vi "TalonMotionMagic.vi"(0 "xMotorControlDevRef":T1={"DeviceStatus"={"status"=FALSE, "code"=0, "source"=""}, "Type"=enum."PWM", "PWM"={"PWM Channel"=enum."Invalid", "DeadBand"={"Name"="", "maxPositivePwm"=0, "minPositivePwm"=0, "centerPwm"=0, "maxNegativePwm"=0, "minNegativePwm"=0, "angularRange"=0}}, "CAN"={"Device Number"=0, "SetOutput VI Ref"=variant, "GetOutput VI Ref"=variant, "Enable VI Ref"=variant, "Disable VI Ref"=variant, "Data"=variant}, "Invert"=FALSE, "DIO PWM"={"PWM \"Enable\" Channel"=enum."Invalid", "DIOChannel"=enum."Invalid", "PWM Rate"=0.0}}, 1 "Boolean Value Inputs":T7, 2 "Numeric Value Inputs":T6, 3 "error in":errorcluster) -> (5 "PhoenixMotorControlDevRef":T1={"DeviceStatus"={"status"=FALSE, "code"=0, "source"=""}, "Type"=enum."PWM", "PWM"={"PWM Channel"=enum."Invalid", "DeadBand"={"Name"="", "maxPositivePwm"=0, "minPositivePwm"=0, "centerPwm"=0, "maxNegativePwm"=0, "minNegativePwm"=0, "angularRange"=0}}, "CAN"={"Device Number"=0, "SetOutput VI Ref"=variant(enum8{"Percent VBus", "Current", "Speed", "Position", "Voltage"} enum."Percent VBus"), "GetOutput VI Ref"=variant(refnum<k1> refnum), "Enable VI Ref"=variant(dbl 12.0), "Disable VI Ref"=variant(enum8{"Percent VBus", "Speed", "Position", "Slave", "Unchanged / Invalid", "Voltage Compensation", "Current", "Motion Profile"} enum."Percent VBus"), "Data"=variant}, "Invert"=FALSE, "DIO PWM"={"PWM \"Enable\" Channel"=enum."Invalid", "DIOChannel"=enum."Invalid", "PWM Rate"=0.0}}, 6 "Graph Output":cluster{"Hood Setpoint":dbl, dbl}, 7 "error out":errorcluster)   [LabVIEW 2020]
uses:
  <vilib>/Rock Robotics/WPI/MotorControl/WPI_MotorControlDeviceRef.ctl
  <vilib>/Rock Robotics/WPI/MotorControl/WPI_MotorControlType.ctl
  <vilib>/Rock Robotics/SystemInterfaces/DIO/FPGA_DIOPWMChannel.ctl
  <vilib>/Rock Robotics/WPI/PWM/WPI_PWMDeadband.ctl
  <vilib>/Rock Robotics/SystemInterfaces/DIO/FPGA_DIOChannel.ctl
  <vilib>/Rock Robotics/WPI/ThirdParty/Phoenix-LabVIEW/Motor Controller/Controls/CTRE_Phoenix_MotorControl_ControlMode.ctl
  <vilib>/Rock Robotics/WPI/ThirdParty/Phoenix-LabVIEW/Motor Controller/Get/CTRE_Phoenix_MotorController_GetSelectedSensorData.vi
  TitanLib/Lib/TitanLib.lvlib
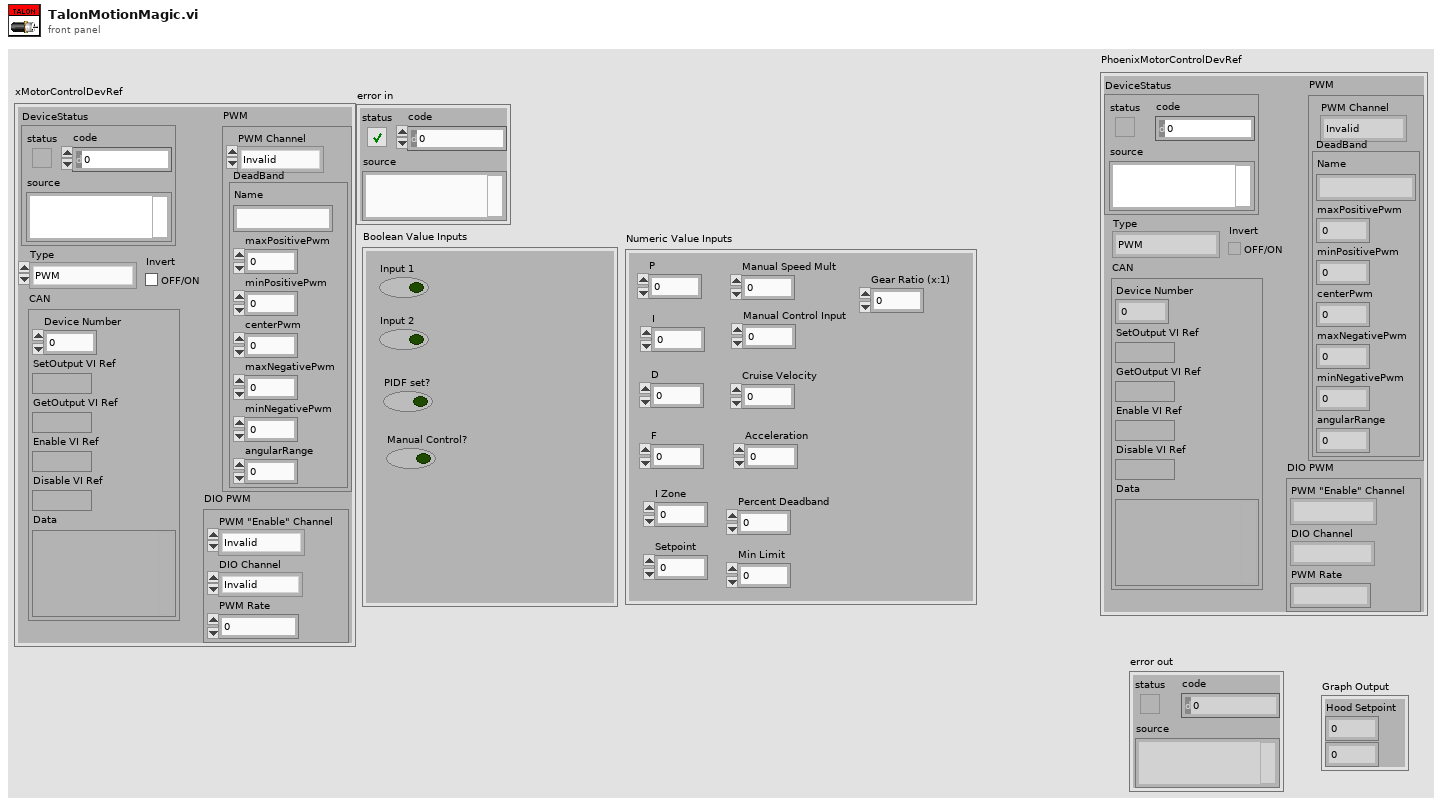
[diagram p1: front panel]
types:
  T1 = typedef "WPI_MotorControlDeviceRef.ctl" = cluster{"DeviceStatus":errorcluster, "Type":T2, "PWM":cluster{"PWM Channel":T3, "DeadBand":T4}, "CAN":cluster{"Device Number":u8, "SetOutput VI Ref":variant, "GetOutput VI Ref":variant, "Enable VI Ref":variant, "Disable VI Ref":variant, "Data":variant}, "Invert":bool, "DIO PWM":cluster{"PWM \"Enable\" Channel":T3, "DIOChannel":T5, "PWM Rate":dbl}}
  T2 = typedef "WPI_MotorControlType.ctl" = enum16{"PWM", "CAN", "DIO PWM"}
  T3 = typedef "FPGA_DIOPWMChannel.ctl" = enum8{"PWM 0", "PWM 1", "PWM 2", "PWM 3", "PWM 4", "PWM 5", "PWM 6", "PWM 7", "PWM 8", "PWM 9", "PWM MXP 0", "PWM MXP 1", "PWM MXP 2", "PWM MXP 3", "PWM MXP 4", "PWM MXP 5", "PWM MXP 6", "PWM MXP 7", "PWM MXP 8", "PWM MXP 9", "Invalid"}
  T4 = typedef "WPI_PWMDeadband.ctl" = cluster{"Name":string, "maxPositivePwm":i32, "minPositivePwm":i32, "centerPwm":i32, "maxNegativePwm":i32, "minNegativePwm":i32, "angularRange":u16}
  T5 = typedef "FPGA_DIOChannel.ctl" = enum8{"DIO 0", "DIO 1", "DIO 2", "DIO 3", "DIO 4", "DIO 5", "DIO 6", "DIO 7", "DIO 8", "DIO 9", "DIO MXP 0", "DIO MXP 1", "DIO MXP 2", "DIO MXP 3", "DIO MXP 4", "DIO MXP 5", "DIO MXP 6", "DIO MXP 7", "DIO MXP 8", "DIO MXP 9", "DIO MXP 10", "DIO MXP 11", "DIO MXP 12", "DIO MXP 13", "DIO MXP 14", "DIO MXP 15", "SPI Port CS1", "SPI Port CS2", "SPI Port CS3", "SPI Port MISO", "SPI Port MOSI", "Invalid"}
  T6 = cluster{"P":dbl, "I":dbl, "D":dbl, "F":dbl, "I Zone":dbl, "Setpoint":dbl, "Manual Speed Mult":dbl, "Manual Control Input":dbl, "Cruise Velocity":i32, "Acceleration":i32, "Percent Deadband":dbl, "Min Limit":dbl, "Gear Ratio (x:1)":dbl}
  T7 = cluster{"Input 1":bool, "Input 2":bool, "PIDF set?":bool, "Manual Control?":bool}
  T8 = typedef "CTRE_Phoenix_MotorControl_ControlMode.ctl" = u16
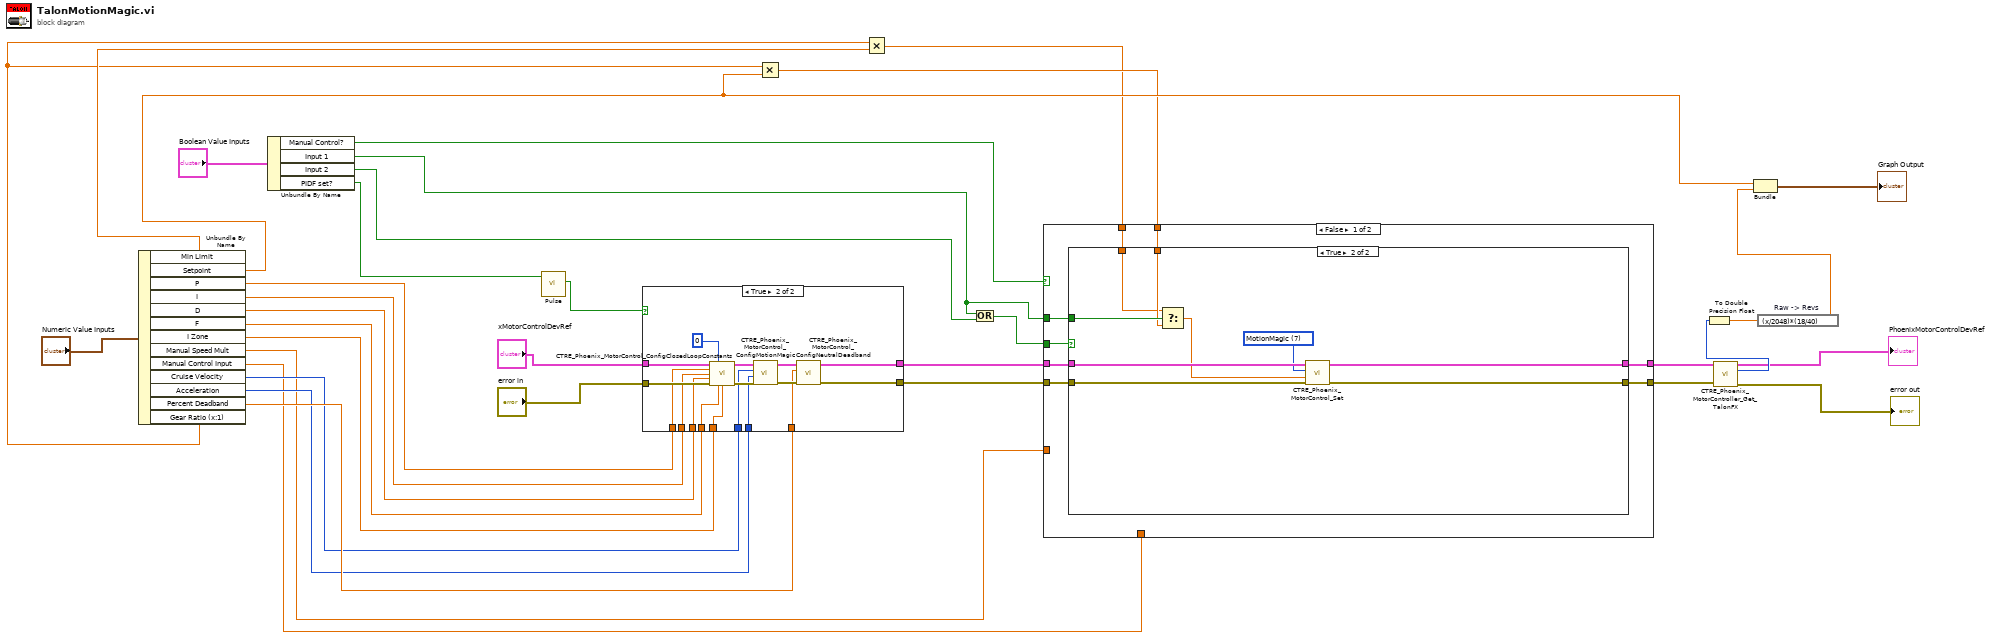
[diagram p0: block diagram]
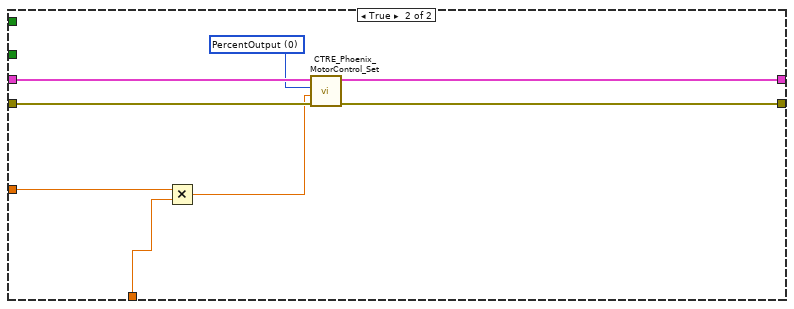
[diagram p3: hidden frame]
diagram:
  n1 = Unbundle By Name("Numeric Value Inputs") -> ("Min Limit"=w4:dbl, "Setpoint"=w5:dbl, "P"=w17:dbl, "I"=w16:dbl, "D"=w15:dbl, "F"=w14:dbl, "I Zone"=w13:dbl, "Manual Speed Mult"=w9:dbl, "Manual Control Input"=w8:dbl, "Cruise Velocity"=w11:i32, "Acceleration"=w10:i32, "Percent Deadband"=w12:dbl, "Gear Ratio (x:1)"=w3:dbl)
  n2 = Unbundle By Name("Boolean Value Inputs") -> ("Manual Control?"=w19:bool, "Input 1"=w20:bool, "Input 2"=w21:bool, "PIDF set?"=w22:bool)
  n3 = call "Pulse.vi"("Input"=w22) -> ("Output"=w26:bool)  [unwired: 10 in]
  n4 = case shown="True" w26 {
    tunnel: "xMotorControlDevRef" -> [w37 w54]
    tunnel: "error in" -> [w36 w53]
    tunnel: w17 -> [_ w52]
    tunnel: w16 -> [_ w51]
    tunnel: w15 -> [_ w50]
    tunnel: w14 -> [_ w49]
    tunnel: w13 -> [_ w48]
    tunnel: w11 -> [_ w45]
    tunnel: w10 -> [_ w44]
    tunnel: w12 -> [_ w41]
    tunnel: [w37 w40] -> w27
    tunnel: [w36 w39] -> w28
    frame False {
    }
    frame True {
      n5 = call <vilib>:"CTRE_Phoenix_MotorControl_ConfigClosedLoopConstants.vi"("PhoenixMotorControlDevRef"=w54, "slotIdx"=0, "P"=w52, "I"=w51, "D"=w50, "error in (no error)"=w53, "F"=w49, "I Zone"=w48) -> ("PhoenixMotorControlDevRef"=w46:T1, "error out"=w47:errorcluster)  [unwired: 6 in]
      n6 = call <vilib>:"CTRE_Phoenix_MotorControl_ConfigMotionMagic.vi"("error in (no error)"=w47, "Acceleration"=w44, "Cruise Velocity"=w45, "PhoenixMotorControlDevRef"=w46) -> ("error out"=w43:errorcluster, "PhoenixMotorControlDevRef"=w42:T1)  [unwired: 6 in]
      n7 = call <vilib>:"CTRE_Phoenix_MotorControl_ConfigNeutralDeadband.vi"("error in (no error)"=w43, "Percent Deadband"=w41, "PhoenixMotorControlDevRef"=w42) -> ("error out"=w39:errorcluster, "PhoenixMotorControlDevRef"=w40:T1)  [unwired: 7 in]
    }
  }
  n8 = Multiply(x=w3, y=w5) -> (x*y=w2:dbl)
  n9 = Multiply(x=w3, y=w4) -> (x*y=w1:dbl)
  n10 = Or(x=w20, y=w21) -> (x .or. y?=w29:bool)
  n11 = case shown="False" w19 {
    tunnel: w27 -> [w62 w81]
    tunnel: w28 -> [w61 w80]
    tunnel: w29 -> [w60 _]
    tunnel: w20 -> [w59 _]
    tunnel: w2 -> [w58 _]
    tunnel: w9 -> [_ w79]
    tunnel: [w57 w76] -> w30
    tunnel: [w56 w75] -> w31
    tunnel: w8 -> [_ w74]
    tunnel: w1 -> [w55 _]
    frame False {
      n12 = case shown="True" w60 {
        tunnel: w62 -> [w64 w73]
        tunnel: w61 -> [w63 w72]
        tunnel: w59 -> [_ w70]
        tunnel: w58 -> [_ w68]
        tunnel: [w64 w67] -> w57
        tunnel: [w63 w66] -> w56
        tunnel: w55 -> [_ w65]
        frame False {
        }
        frame True {
          w71 = T8 7 items=["PercentOutput"=0, "Position"=1, "Velocity"=2, "Current"=3, "Follower"=5, "MotionProfile"=6, "MotionMagic"=7, "MotionProfileArc"=10, "Disabled"=15] ("Control Mode")
          n13 = Select(t=w65, s=w70, f=w68) -> (s? t:f=w69:dbl)
          n14 = call <vilib>:"CTRE_Phoenix_MotorControl_Set.vi"("error in (no error)"=w72, "Output"=w69, "Control Mode"=w71, "PhoenixMotorControlDevRef"=w73) -> ("error out"=w66:errorcluster, "PhoenixMotorControlDevRef"=w67:T1)  [unwired: 6 in]
        }
      }
    }
    frame True {
      w77 = T8 0 items=["PercentOutput"=0, "Position"=1, "Velocity"=2, "Current"=3, "Follower"=5, "MotionProfile"=6, "MotionMagic"=7, "MotionProfileArc"=10, "Disabled"=15] ("Control Mode")
      n15 = Multiply(x=w79, y=w74) -> (x*y=w78:dbl)
      n16 = call <vilib>:"CTRE_Phoenix_MotorControl_Set.vi"("error in (no error)"=w80, "Output"=w78, "Control Mode"=w77, "PhoenixMotorControlDevRef"=w81) -> ("error out"=w75:errorcluster, "PhoenixMotorControlDevRef"=w76:T1)  [unwired: 6 in]
    }
  }
  n17 = call-poly <vilib>:"CTRE_Phoenix_MotorController_Get_TalonFX.vi"("PhoenixMotorControlDevRef"=w30, "error in"=w31) -> ("PhoenixMotorControlDevRef"=→"PhoenixMotorControlDevRef":T1, "Position (Raw Sensor Units)"=w32:i32, "error out"=→"error out":errorcluster)  [unwired: 10 in, 1 out]
  n18 = To Double Precision Float(number=w32) -> (double precision float=w33:dbl)
  n19 = expression code="(x/2048)*(18/40)" "Raw -> Revs"(w33) -> (w34:dbl)
  n20 = Bundle("Setpoint"=w5, w34) -> (→"Graph Output":cluster{"Setpoint":dbl, dbl})  [unwired: 1 in]
